vi "Launcher.vi"() -> ()   [LabVIEW 2014, in "HIJ Vision Camera App w Timer.lvlib"]
uses:
  HIJ Vision Camera App w Timer.lvlib
  <vilib>/userdefined/High Color/IMAQdx.ctl
  HIJ Vision Camera App w Timer/HIJ Vision Camera App w Timer.lvclass
  HIJ Vision Camera App w Timer/HIJ Vision Camera App w Timer.lvclass/HIJ Vision Camera App w Timer.ctl
  Shared Code/Viewable Actor/ViewableActor Messages/Set Window Titel Msg/Set Window Titel Msg.lvclass/Set Window Titel Msg.ctl
  <vilib>/ActorFramework/Message Enqueuer/Message Enqueuer.lvclass/Message Enqueuer.ctl
  HIJ Vision Camera App w Timer/Write Camera.vi
  HIJ Vision Camera App w Timer/Write Config Dir.vi
  HIJ Vision Camera App w Timer/Write Work Dir.vi
  HIJ Vision Camera App w Timer/Write Shot Rate.vi
  <vilib>/ActorFramework/Message Enqueuer/Enqueue.vi
  <vilib>/Utility/config.llb/Read Key (Path).vi
  <vilib>/Utility/config.llb/Read Key (String).vi
  <vilib>/Utility/config.llb/Read Key (Double).vi
  <vilib>/ActorFramework/Message Priority Queue/Priority Enqueue.vi
  <vilib>/Utility/config.llb/Write Key (Path).vi
  <vilib>/Utility/config.llb/Write Key (String).vi
  <vilib>/Utility/config.llb/Write Key (Double).vi
  Shared Code/Viewable Actor/ViewableActor Messages/Set Window Titel Msg/Set Window Titel Msg.lvclass
  <vilib>/ActorFramework/Actor/Actor.lvclass
  <vilib>/Utility/config.llb/NI_LVConfig.lvlib
panel:
  in  "Shot Rate":dbl=10.0 format="%#_13g"
  in  "UI Cnfg":path
  in  "CLine Parameter":string
  in  "RUN_STOP":bool=TRUE
  in  "Start WorkDir":path=path "C:/Users/user/Desktop/test/WorkDir"
  in  "Start ConfigDir":path=path "C:/Users/user/Desktop/test/ConfigDir"
  in  "Start Camera":T1="TestCam"
  out "error out":errorcluster
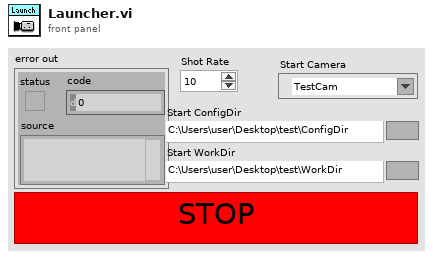
[diagram p1: front panel]
types:
  T1 = typedef "IMAQdx.ctl" = refnum<k21>
  T2 = typedef "NI_LVConfig.lvlib/Config Data RefNum.ctl" = refnum<k1>
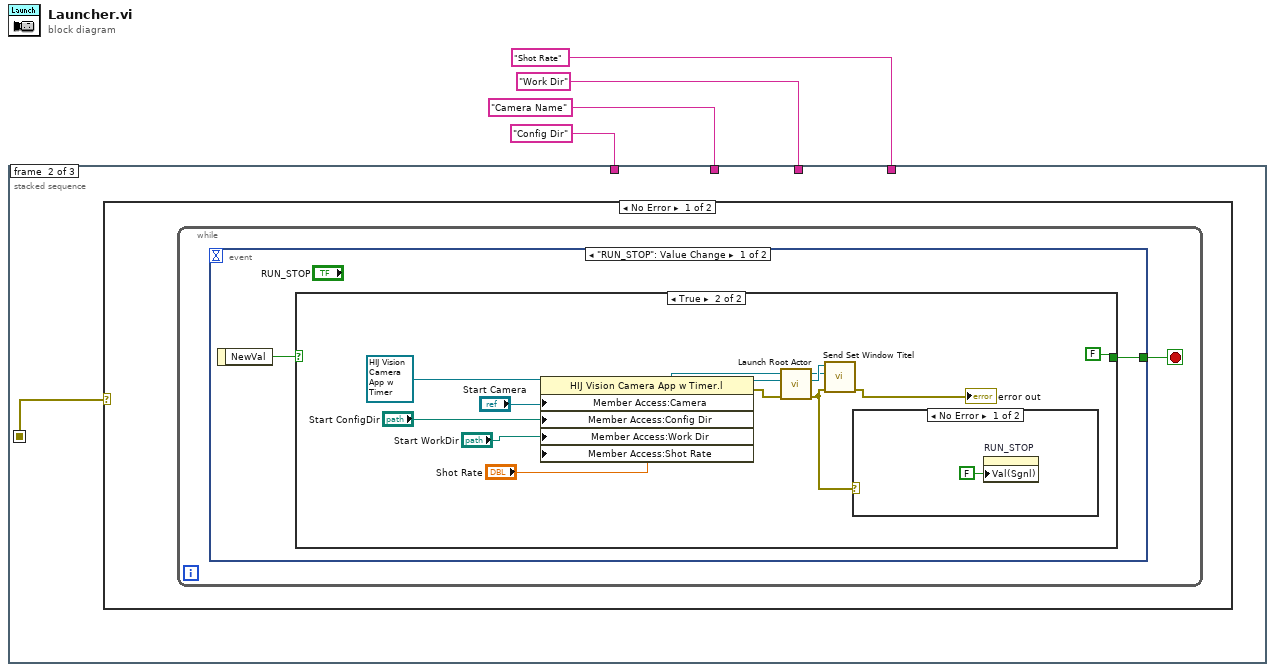
[diagram p0: block diagram]
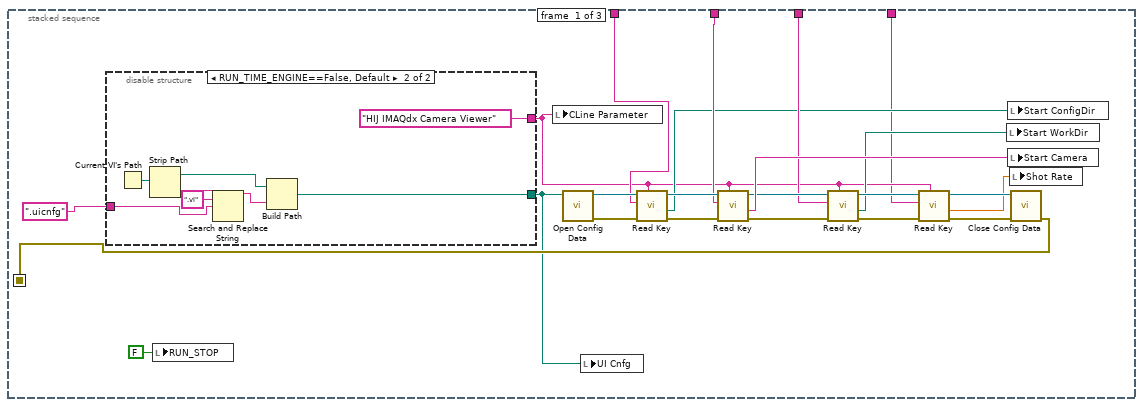
[diagram p2: hidden frame]
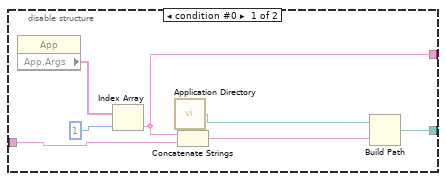
[diagram p3: hidden frame]
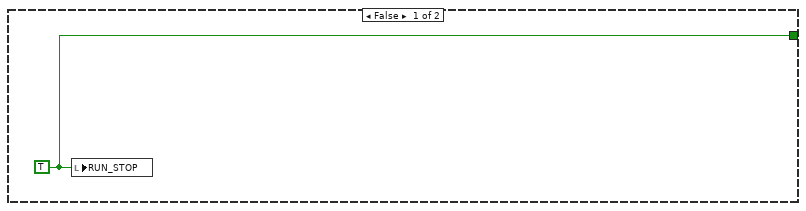
[diagram p4: hidden frame]
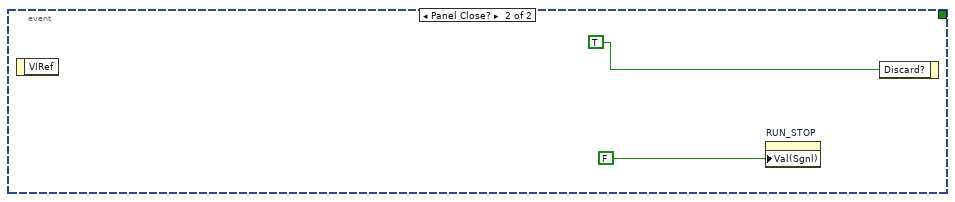
[diagram p6: hidden frame]
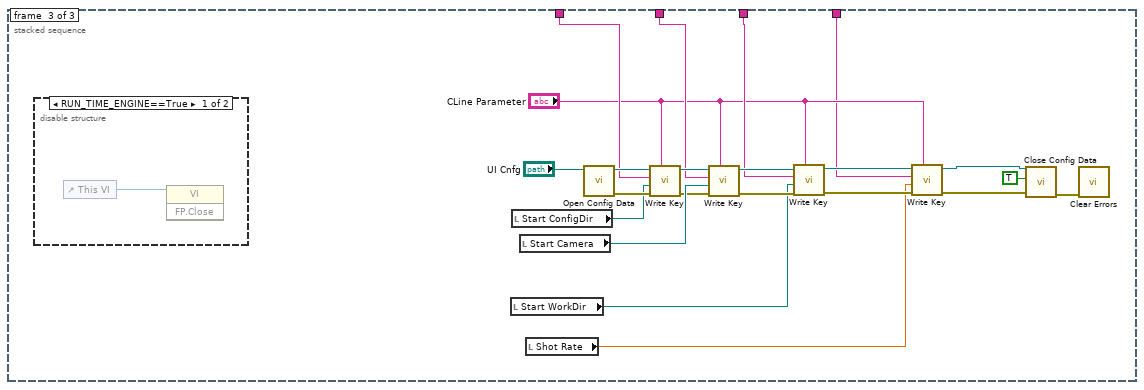
[diagram p8: hidden frame]
diagram:
  n1 = stacked-sequence {
    seq-local: [w20 _ _] -> [_ w43 _]
    tunnel: "Camera Name" ("key") -> [w22 _ w79]
    tunnel: "Config Dir" ("key") -> [w21 _ w80]
    tunnel: "Work Dir" ("key") -> [w13 _ w68]
    tunnel: "Shot Rate" ("key") -> [w5 _ w63]
    frame #0 {
      n2 = disable-structure shown="RUN_TIME_ENGINE==False, Default" {
        disable-tunnel: [w30 w36] -> w18
        disable-tunnel: ".uicnfg" ("string") -> [w29 w39]
        disable-tunnel: [w28 "HIJ IMAQdx Camera Viewer"] -> w9
        frame condition #0 {
          n3 = property class="App"() -> ("App.Args"=w34:string[])  [unwired: 2 in, 2 out]
          n4 = Index Array(array=w34, index=1) -> (element=w28:string)
          n5 = call <vilib>:"Application Directory.vi"() -> ("Application Directory"=w32:path)
          n6 = Concatenate Strings(w28, w29) -> (w31:string)
          n7 = Build Path(base path=w32, name or relative path=w31) -> (appended path=w30:path)
        }
        frame condition #1 (active) {
          n8 = Current VI's Path() -> (path=w42:path)
          n9 = Strip Path(path=w42) -> (stripped path=w37:path, name=w41:string)
          n10 = Search and Replace String(input string=w41, search string=".vi", replace string=w39) -> (result string=w38:string)  [unwired: 5 in, 3 out]
          n11 = Build Path(base path=w37, name or relative path=w38) -> (appended path=w36:path)
        }
      }
      n12 = local write "RUN_STOP"(FALSE ("RUN_STOP")) -> ()
      n13 = local write "CLine Parameter"(w9) -> ()
      n14 = call <vilib>:"Open Config Data.vi"("configuration file path"=w18) -> ("error out"=w24:errorcluster, "refnum"=w23:T2)  [unwired: 8 in, 1 out]
      n15 = local write "UI Cnfg"(w18) -> ()
      n16 = call-poly <vilib>:"Read Key.vi"("section"=w9, "error in (no error)"=w24, "key"=w21, "refnum"=w23) -> ("error out"=w25:errorcluster, "value"=w11:path, "refnum out"=w26:T2)  [unwired: 4 in, 1 out]
      n17 = call-poly <vilib>:"Read Key.vi"("section"=w9, "error in (no error)"=w25, "key"=w22, "refnum"=w26) -> ("error out"=w16:errorcluster, "value"=w17:string, "refnum out"=w15:T2)  [unwired: 4 in, 1 out]
      n18 = call-poly <vilib>:"Read Key.vi"("section"=w9, "error in (no error)"=w16, "key"=w13, "refnum"=w15) -> ("error out"=w7:errorcluster, "value"=w12:path, "refnum out"=w14:T2)  [unwired: 4 in, 1 out]
      n19 = call-poly <vilib>:"Read Key.vi"("section"=w9, "error in (no error)"=w7, "key"=w5, "refnum"=w14) -> ("error out"=w6:errorcluster, "value"=w8:dbl, "refnum out"=w10:T2)  [unwired: 4 in, 1 out]
      n20 = local write "Start WorkDir"(w12) -> ()
      n21 = local write "Start ConfigDir"(w11) -> ()
      n22 = local write "Start Camera"(w17) -> ()
      n23 = local write "Shot Rate"(w8) -> ()
      n24 = call <vilib>:"Close Config Data.vi"("error in (no error)"=w6, "refnum"=w10) -> ("error out"=w20:errorcluster)  [unwired: 8 in, 1 out]
    }
    frame #1 {
      n25 = case shown="No Error" w43 {
        frame No Error {
          n26 = while {
            stop <- w44 stop-if-true
            n27 = event shown="[0] \"RUN_STOP\": Value Change" {
              selector: _ -> [_ _]
              dyn-events: _ -> [_ _]
              timeout: _ -> [_ _]
              tunnel: [w46 _] -> w44
              event "RUN_STOP": Value Change {
                n28 = event-data() -> ("NewVal"=w45:bool)  [unwired: 1 in]
                n29 = case shown="True" w45 {
                  tunnel: [w47 FALSE] -> w46
                  frame False {
                    w47 = TRUE ("RUN_STOP")
                    n30 = local write "RUN_STOP"(w47) -> ()
                  }
                  frame True {
                    n31 = property class="HIJ Vision Camera App w Timer.l"(reference=refnum<class "HIJ Vision Camera App w Timer.lvclass"> refnum ("Launch IMAQ Display.lvlib:Launch IMAQ Display.lvclass"), "Member Access:Camera"="Start Camera", "Member Access:Config Dir"="Start ConfigDir", "Member Access:Work Dir"="Start WorkDir", "Member Access:Shot Rate"="Shot Rate") -> (reference out=w54:refnum<class "HIJ Vision Camera App w Timer.lvclass">, error out=w55:errorcluster)  [unwired: 1 in]
                    n32 = call <vilib>:"Launch Root Actor.vi"("error in (no error)"=w55, "Actor"=w54) -> ("error out"=w52:errorcluster, "Actor's Enqueuer"=w51:refnum<class "Message Enqueuer.lvclass">)  [unwired: 8 in]
                    n33 = call "Send Set Window Titel.vi"("error in (no error)"=w52, "Title"="Start Camera", "Message Enqueuer"=w51) -> ("error out"=→"error out":errorcluster)  [unwired: 7 in, 1 out]
                    n34 = case shown="No Error" w52 {
                      frame No Error {
                        n35 = property on="RUN_STOP" class="Bool (strict)"("Val(Sgnl)"=FALSE ("Value (Signaling)")) -> ()  [unwired: 2 in, 2 out]
                      }
                      frame Error {
                      }
                    }
                  }
                }
              }
              event Panel Close? {
                n36 = event-data() -> ()  [unwired: 1 in, 1 out]
                n37 = property on="RUN_STOP" class="Bool (strict)"("Val(Sgnl)"=FALSE ("Value (Signaling)")) -> ()  [unwired: 2 in, 2 out]
                n38 = event-data("Discard?"=TRUE) -> ()  [unwired: 1 in, 1 out]
              }
            }
          }
        }
        frame Error {
        }
      }
    }
    frame #2 {
      n39 = disable-structure shown="RUN_TIME_ENGINE==True" {
        frame condition #0 {
          n40 = control-ref of="This VI"() -> (w84:refnum<vi>)
          n41 = invoke class="VI" method="FP.Close"(reference=w84) -> ()  [unwired: 2 in, 3 out]
        }
        frame condition #1 (active) {
        }
      }
      n42 = local read "Start WorkDir"() -> (w69:path)
      n43 = local read "Start ConfigDir"() -> (w73:path)
      n44 = local read "Start Camera"() -> (w78:T1)
      n45 = local read "Shot Rate"() -> (w62:dbl)
      n46 = call <vilib>:"Open Config Data.vi"("configuration file path"="UI Cnfg") -> ("error out"=w77:errorcluster, "refnum"=w82:T2)  [unwired: 8 in, 1 out]
      n47 = call-poly <vilib>:"Write Key.vi"("section"="CLine Parameter", "error in (no error)"=w77, "value"=w73, "key"=w80, "refnum"=w82) -> ("error out"=w76:errorcluster, "refnum out"=w83:T2)  [unwired: 4 in, 1 out]
      n48 = call-poly <vilib>:"Write Key.vi"("section"="CLine Parameter", "error in (no error)"=w76, "value"=w78, "key"=w79, "refnum"=w83) -> ("error out"=w71:errorcluster, "refnum out"=w72:T2)  [unwired: 4 in, 1 out]
      n49 = call-poly <vilib>:"Write Key.vi"("section"="CLine Parameter", "error in (no error)"=w71, "value"=w69, "key"=w68, "refnum"=w72) -> ("error out"=w66:errorcluster, "refnum out"=w70:T2)  [unwired: 4 in, 1 out]
      n50 = call-poly <vilib>:"Write Key.vi"("section"="CLine Parameter", "error in (no error)"=w66, "value"=w62, "key"=w63, "refnum"=w70) -> ("error out"=w65:errorcluster, "refnum out"=w67:T2)  [unwired: 4 in, 1 out]
      n51 = call <vilib>:"Close Config Data.vi"("error in (no error)"=w65, "write file if changed (T)"=TRUE, "refnum"=w67) -> ("error out"=w75:errorcluster)  [unwired: 7 in, 1 out]
      n52 = call <vilib>:"Clear Errors.vi"("error in (no error)"=w75) -> ()  [unwired: 5 in, 2 out]
    }
  }
